vi "Main.vi"(11 "Module Admin":refnum<class "Delacor_lib_QMH_Module Admin.lvclass">) -> ()   [LabVIEW 2024, in "MoneyControl.lvlib"]
doc: "This template is based off of the Queued Message Handler design pattern and the Queued Message Handler project template that ships with LabVIEW.\n\nThe main difference is that the queue is private to this module and communication between modules is performed via Broadcast and Request events.\n\nRequest events are wrapped in public API methods and are handled in the Event Handling Loop (EHL) of this VI. Any module can register for Broadcast events sent by this module. The EHL generates messages based on user interface actions.\n\nThe Message Handling Loop (MHL) processes messages generated by the EHL, or by other messages. The messages are string values, so new messages can be added easily to the Message Cases case structure in the MHL. Each message cluster can also provide an optional value for Message Data, which is a variant that can be converted to whatever message-specific data is required.\n_____\nBased on DQMH Dev Tools: Project Template 7.1.0.1503."
uses:
  MoneyControl.lvlib
  <vilib>/Delacor/Delacor QMH/Libraries/Module Admin_class/Delacor_lib_QMH_Module Admin.lvclass
  Module Data--cluster.ctl
  Incrementa Credito Argument--cluster.ctl
  <vilib>/Delacor/Delacor QMH/Libraries/Message Queue_class/Delacor_lib_QMH_Message Queue.lvclass/Delacor_lib_QMH_Message Queue.ctl
  Stop Argument--cluster.ctl
  <vilib>/Delacor/Delacor QMH/Libraries/Module Admin_class/Delacor_lib_QMH_Module Admin.lvclass/Delacor_lib_QMH_Module Admin.ctl
  Draw FP in Subpanel Argument--cluster.ctl
  Remove From Subpanel Argument--cluster.ctl
  Devuelve dinero Argument--cluster.ctl
  Entrega Cambio Argument--cluster.ctl
  consulta credito Argument--cluster.ctl
  consulta credito (Reply Payload)--cluster.ctl
  <vilib>/Delacor/Delacor QMH/Libraries/Message Queue_class/Delacor_lib_QMH_Enqueue Message (Single).vi
  <vilib>/Delacor/Delacor QMH/Libraries/Module Admin_class/Delacor_lib_QMH_Get External Launch.vi
  <vilib>/Delacor/Delacor QMH/Libraries/Message Queue_class/Delacor_lib_QMH_Message Queue.lvclass
panel:
  in  "1":bool
  out "Status":string
  in  "2":bool
  out "error out":errorcluster
  in  "5":bool
  in  "10":bool
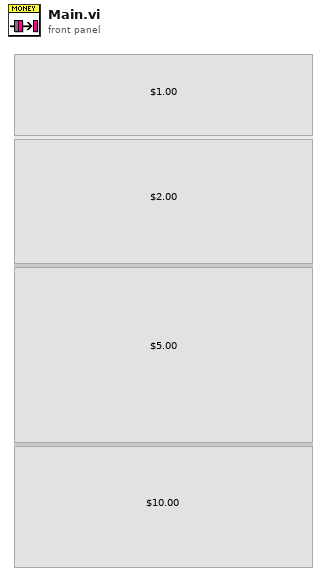
[diagram p1: front panel]
types:
  T1 = typedef "MoneyControl.lvlib/Request Events--cluster.ctl" = cluster{"Stop Module":refnum<user-event>, "Show Panel":refnum<user-event>, "Hide Panel":refnum<user-event>, "Get Module Execution Status":refnum<user-event>, "Show Diagram":refnum<user-event>, "Draw FP in Subpanel":refnum<user-event>, "Remove From Subpanel":refnum<user-event>, "Incrementa Credito":refnum<user-event>, "Devuelve dinero":refnum<user-event>, "Entrega Cambio":refnum<user-event>, "consulta credito":refnum<user-event>}
  T2 = typedef "MoneyControl.lvlib/Module Data--cluster.ctl" = cluster{"Status":string, "Sub Panel":refnum<vi>, "Credito":dbl}
  T3 = typedef "MoneyControl.lvlib/Incrementa Credito Argument--cluster.ctl" = cluster{"Money Value":dbl}
  T4 = enum32{"invalid lock state", "Not Locked", "Locked (No Password)", "Password-protected"}
  T5 = typedef "MoneyControl.lvlib/Stop Argument--cluster.ctl" = cluster{"Origin":string, "Exit via Stop Module Req?":bool, "Wait for Module to stop?":bool}
  T6 = typedef "MoneyControl.lvlib/Draw FP in Subpanel Argument--cluster.ctl" = cluster{"Sub Panel":refnum<vi>}
  T7 = typedef "MoneyControl.lvlib/Remove From Subpanel Argument--cluster.ctl" = cluster{"Boolean":bool}
  T8 = typedef "MoneyControl.lvlib/Devuelve dinero Argument--cluster.ctl" = cluster{"Boolean":bool}
  T9 = typedef "MoneyControl.lvlib/Entrega Cambio Argument--cluster.ctl" = cluster{"Valor Producto":dbl}
  T10 = typedef "MoneyControl.lvlib/consulta credito Argument--cluster.ctl" = cluster{"Wait Notifier":refnum<notifier>, "wait for reply":bool}
  T11 = enum32{"Invalid", "Standard", "Closed", "Hidden", "Minimized", "Maximized"}
  T12 = typedef "MoneyControl.lvlib/consulta credito (Reply Payload)--cluster.ctl" = cluster{"Credito Actual":dbl, "error":errorcluster}
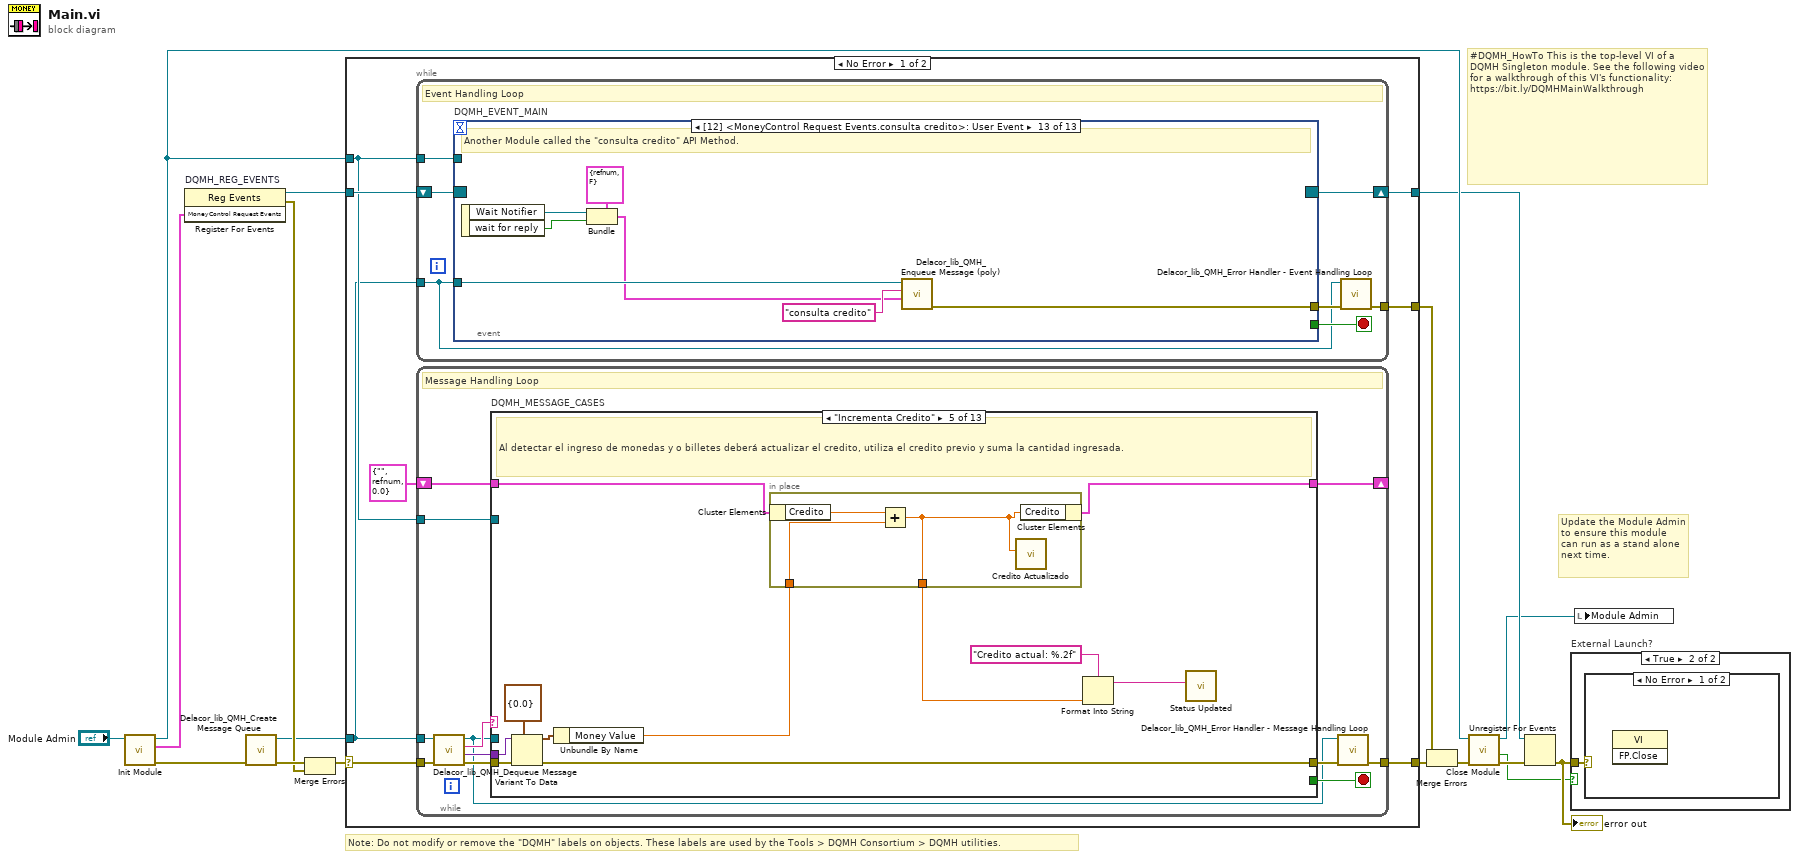
[diagram p0: block diagram]
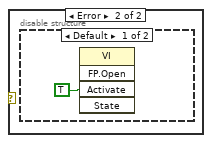
[diagram p3: hidden frame]
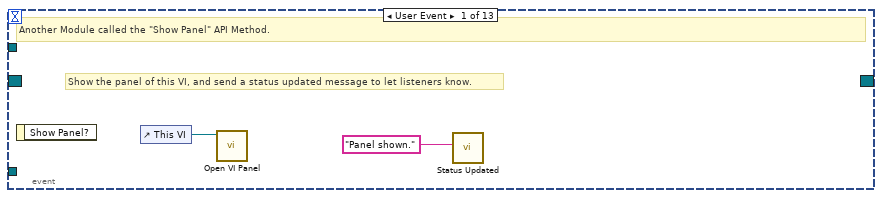
[diagram p5: hidden frame]
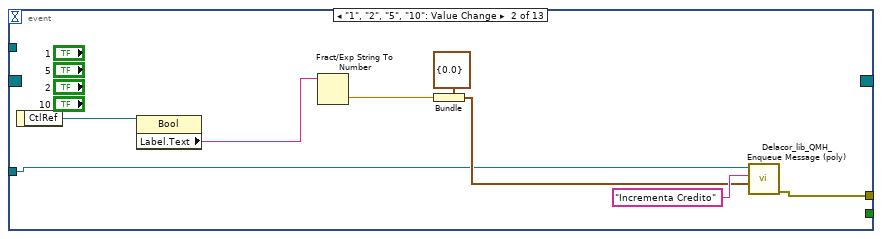
[diagram p6: hidden frame]
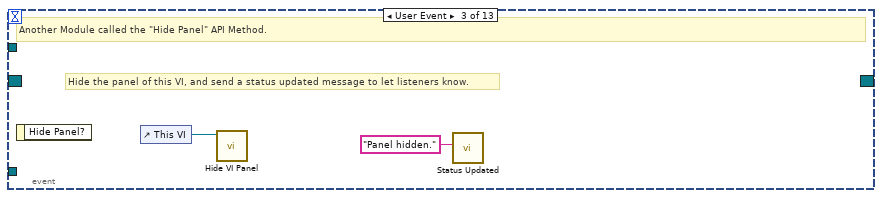
[diagram p7: hidden frame]
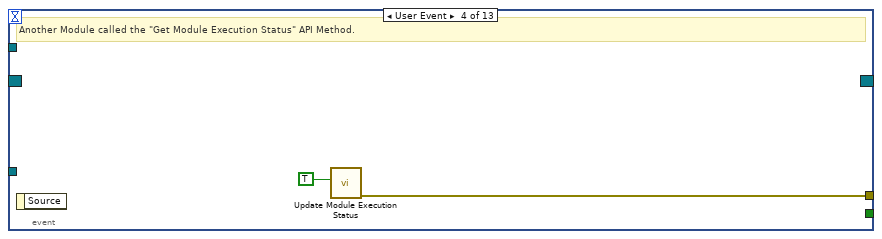
[diagram p8: hidden frame]
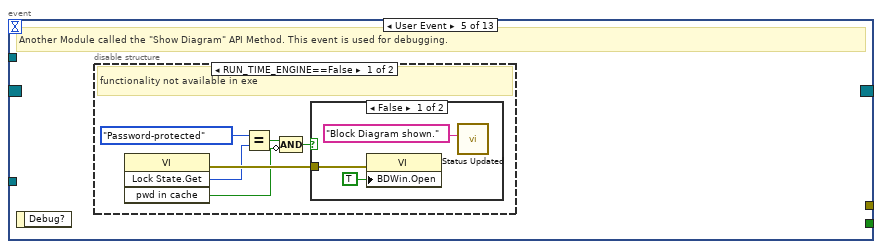
[diagram p9: hidden frame]
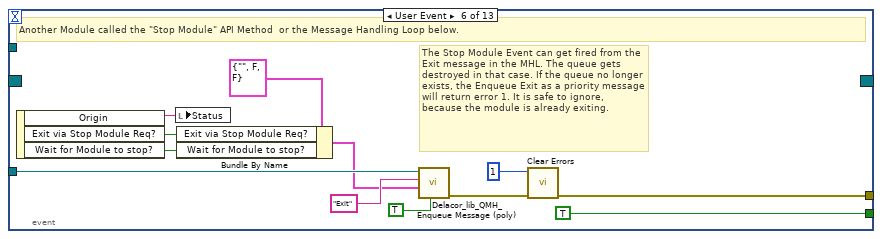
[diagram p12: hidden frame]
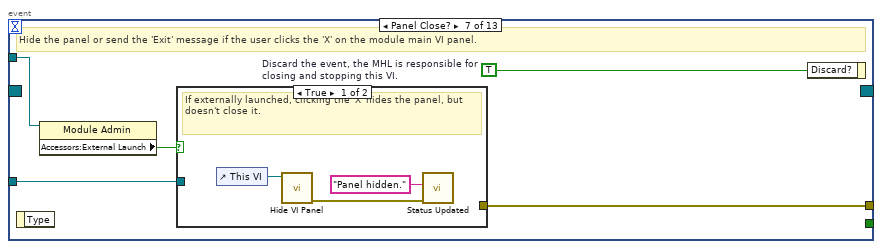
[diagram p13: hidden frame]
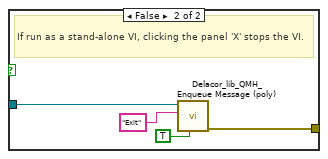
[diagram p14: hidden frame]
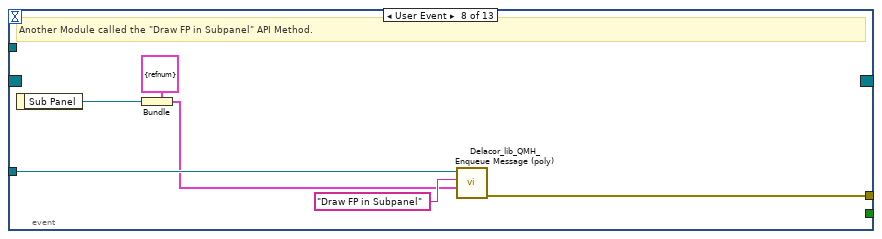
[diagram p15: hidden frame]
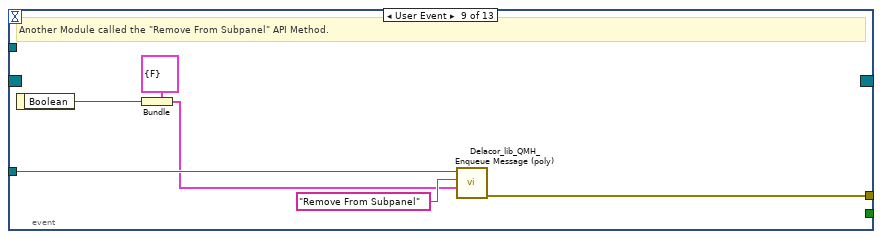
[diagram p16: hidden frame]
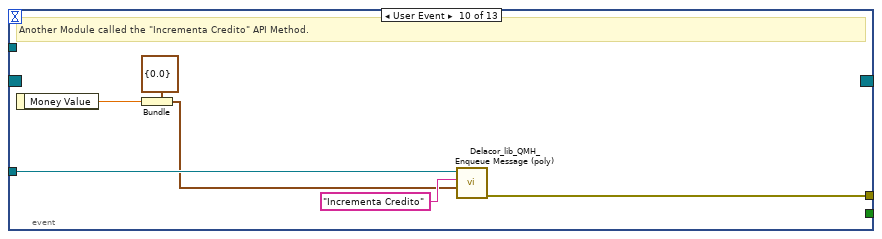
[diagram p17: hidden frame]
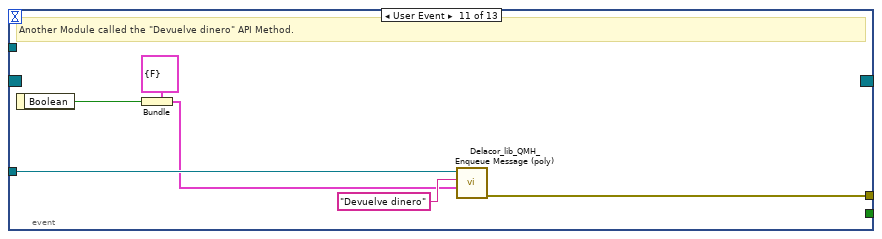
[diagram p18: hidden frame]
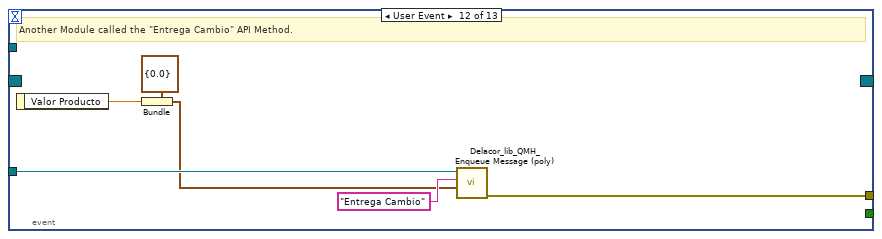
[diagram p19: hidden frame]
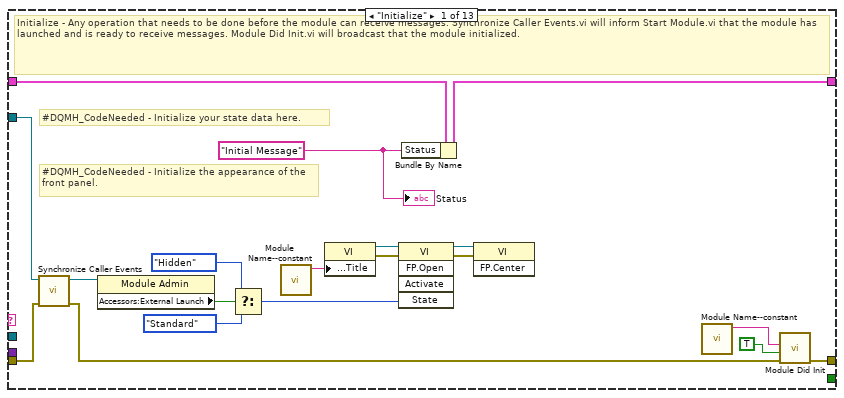
[diagram p20: hidden frame]
diagram:
  # "#DQMH_HowTo This is the top-level VI of a DQMH Singleton module. See the following video for a walkthrough of this VI's functionality: https://bit.ly/DQMHMainWalkthrough"
  # "Note: Do not modify or remove the \"DQMH\" labels on objects. These labels are used by the Tools > DQMH Consortium > DQMH utilities."
  # "Update the Module Admin to ensure this module can run as a stand alone next time."
  n1 = call "Init Module.vi"("Singleton Module Admin in"="Module Admin") -> ("error out"=w16:errorcluster, "MoneyControl Request Events"=w5:T1, "Singleton Module Admin out"=w8:refnum<class "Delacor_lib_QMH_Module Admin.lvclass">)  [unwired: 8 in]
  n2 = register-events "DQMH_REG_EVENTS"(w5) -> (reference out=w6:refnum<event-registration>, error out=w9:errorcluster)  [unwired: 2 in]
  n3 = call <vilib>:"Delacor_lib_QMH_Create Message Queue.vi"("error in"=w16) -> ("error out"=w11:errorcluster, "Message Queue"=w4:refnum<class "Delacor_lib_QMH_Message Queue.lvclass">)  [unwired: 9 in]
  n4 = Merge Errors(w11, w9) -> (w10:errorcluster)
  n5 = case shown="No Error" w10 {
    selector: w10 -> [w23 w296]
    tunnel: [w25 w295] -> w17
    tunnel: [w22 w294] -> w7
    tunnel: w6 -> [w20 w294]
    tunnel: w4 -> [w18 w289]
    tunnel: [w24 _] -> w14
    tunnel: w8 -> [w19 w290]
    frame No Error {
      n6 = while {
        tunnel: w18 -> [w26]
        shift-right: [w29] -> w22
        shift-left: w20 -> [w30]
        tunnel: [w31] -> w24
        tunnel: w19 -> [w27]
        stop <- w28 stop-if-true
        # "Event Handling Loop"
        n7 = event "DQMH_EVENT_MAIN" shown="[12] <MoneyControl Request Events.consulta credito>: User Event" {
          selector: w30 -> [_ _ _ _ _ _ _ _ _ _ _ _ _]
          dyn-events: [_ _ _ _ _ _ _ _ _ _ _ _ _] -> w29
          timeout: _ -> [_ _ _ _ _ _ _ _ _ _ _ _ _]
          tunnel: [_ _ _ _ _ TRUE ("Discard?") _ _ _ _ _ _ _] -> w28
          tunnel: w26 -> [_ w37 _ _ _ w63 w70 w84 w90 w97 w103 w109 w116]
          tunnel: [_ w38 _ w46 _ w66 w72 w85 w91 w92 w98 w104 w110] -> w32
          tunnel: w27 -> [_ _ _ _ _ _ w69 _ _ _ _ _ _]
          event User Event {
            # "Show the panel of this VI, and send a status updated message to let listeners know."
            # "Another Module called the \"Show Panel\" API Method."
            n8 = event-data() -> ()  [unwired: 1 in, 1 out]
            n9 = control-ref of="This VI"() -> (w34:refnum<vi>)
            n10 = call "Open VI Panel.vi"("VI"=w34) -> ()  [unwired: 10 in, 1 out]
            n11 = call "Status Updated.vi"("Status"="Panel shown." ("format string")) -> ()  [unwired: 10 in, 1 out]
          }
          event "1", "2", "5", "10": Value Change {
            n12 = event-data() -> ("CtlRef"=w42:refnum<vi>)  [unwired: 1 in]
            n13 = property class="Bool"(reference=w42) -> ("Label.Text"=w36:string)  [unwired: 1 in, 2 out]
            n14 = Fract/Exp String To Number(string=w36) -> (number=w35:dbl)  [unwired: 3 in, 1 out]
            n15 = Bundle(cluster=T3 {"Money Value"=0.0} ("Incrementa Credito Argument"), "Money Value"=w35) -> (w39:T3)
            n16 = call-poly <vilib>:"Delacor_lib_QMH_Enqueue Message (poly).vi"("Message Data"=w39, "Message"="Incrementa Credito", "Message Queue in"=w37) -> ("error out"=w38:errorcluster)  [unwired: 7 in, 1 out]
          }
          event User Event {
            # "Hide the panel of this VI, and send a status updated message to let listeners know."
            # "Another Module called the \"Hide Panel\" API Method."
            n17 = event-data() -> ()  [unwired: 1 in, 1 out]
            n18 = control-ref of="This VI"() -> (w44:refnum<vi>)
            n19 = call "Hide VI Panel.vi"("VI"=w44) -> ()  [unwired: 10 in, 1 out]
            n20 = call "Status Updated.vi"("Status"="Panel hidden." ("format string")) -> ()  [unwired: 10 in, 1 out]
          }
          event User Event {
            # "Another Module called the \"Get Module Execution Status\" API Method."
            n21 = event-data() -> ()  [unwired: 1 in, 1 out]
            n22 = call "Update Module Execution Status.vi"("Running?"=TRUE) -> ("error out"=w46:errorcluster)  [unwired: 10 in]
          }
          event User Event {
            # "Another Module called the \"Show Diagram\" API Method. This event is used for debugging."
            n23 = event-data() -> ()  [unwired: 1 in, 1 out]
            n24 = disable-structure shown="RUN_TIME_ENGINE==False" {
              frame condition #0 (active) {
                # "functionality not available in exe"
                n25 = invoke on="Invoke Node" class="VI" method="Lock State.Get"() -> (error out=w52:errorcluster, "Get Lock State"=w51:T4, "pwd in cache"=w48:bool)  [unwired: 4 in, 1 out]
                n26 = Equal?(x=T4."Password-protected", y=w51) -> (x = y?=w49:bool)
                n27 = Compound Arithmetic op=AND(w49, invert w48) -> (w47:bool)
                n28 = case shown="False" w47 {
                  tunnel: w52 -> [w55 _]
                  frame False {
                    n29 = property on="Property Node" class="VI"(error in=w55, "BDWin.Open"=TRUE ("Block Diagram Window:Open")) -> ()  [unwired: 1 in, 2 out]
                    n30 = call "Status Updated.vi"("Status"="Block Diagram shown." ("format string")) -> ()  [unwired: 10 in, 1 out]
                  }
                  frame True {
                    # "Password-protected VI, and the password is not in the cache. Do not show the diagram."
                  }
                }
              }
              frame condition #1 {
              }
            }
          }
          event User Event {
            # "The Stop Module Event can get fired from the Exit message in the MHL. The queue gets destroyed in that case. If the queue no longer exists, the Enqueue Exit as a priority message will return error 1. It is safe to ignore, because the module is already exiting."
            # "Another Module called the \"Stop Module\" API Method  or the Message Handling Loop below."
            n31 = event-data() -> ("Origin"=w62:string, "Exit via Stop Module Req?"=w58:bool, "Wait for Module to stop?"=w57:bool)  [unwired: 1 in]
            n32 = local write "Status"(w62) -> ()
            n33 = Bundle By Name(cluster=T5 {"Origin"="", "Exit via Stop Module Req?"=FALSE, "Wait for Module to stop?"=FALSE} ("Stop Argument"), "Exit via Stop Module Req?"=w58, "Wait for Module to stop?"=w57) -> (w56:T5)
            n34 = call-poly <vilib>:"Delacor_lib_QMH_Enqueue Message (poly).vi"("Priority Message? (F)"=TRUE, "Message Data"=w56, "Message"="Exit", "Message Queue in"=w63) -> ("error out"=w67:errorcluster)  [unwired: 6 in, 1 out]
            n35 = call <vilib>:"Clear Errors.vi"("error in (no error)"=w67, "specific error code to clear (0: all)"=1) -> ("error out"=w66:errorcluster)  [unwired: 4 in, 1 out]
          }
          event Panel Close? {
            w71 = TRUE  # Discard the event, the MHL is responsible for closing and stopping this VI.
            # "Hide the panel or send the 'Exit' message if the user clicks the 'X' on the module main VI panel."
            n36 = event-data() -> ()  [unwired: 1 in, 1 out]
            n37 = property on="Property Node" class="Module Admin"(reference=w69) -> ("Accessors:External Launch"=w68:bool)  [unwired: 1 in, 2 out]
            n38 = case shown="True" w68 {
              tunnel: w70 -> [_ w78]
              tunnel: [_ w79] -> w72
              frame True {
                # "If externally launched, clicking the 'X' hides the panel, but doesn't close it."
                n39 = control-ref of="This VI"() -> (w74:refnum<vi>)
                n40 = call "Hide VI Panel.vi"("VI"=w74) -> ("error out"=w75:errorcluster)  [unwired: 10 in]
                n41 = call "Status Updated.vi"("error in"=w75, "Status"="Panel hidden." ("format string")) -> ()  [unwired: 9 in, 1 out]
              }
              frame False {
                # "If run as a stand-alone VI, clicking the panel 'X' stops the VI."
                n42 = call-poly <vilib>:"Delacor_lib_QMH_Enqueue Message (poly).vi"("Priority Message? (F)"=TRUE, "Message"="Exit", "Message Queue in"=w78) -> ("error out"=w79:errorcluster)  [unwired: 7 in, 1 out]
              }
            }
            n43 = event-data ("Event Filter Node")("Discard?"=w71) -> ()  [unwired: 1 in, 1 out]
          }
          event User Event {
            # "Another Module called the \"Draw FP in Subpanel\" API Method."
            n44 = event-data() -> ("Sub Panel"=w80:refnum<vi>)  [unwired: 1 in]
            n45 = Bundle(cluster=T6 {"Sub Panel"=refnum} ("Draw FP in Subpanel Argument"), "Sub Panel"=w80) -> (w81:T6)
            n46 = call-poly <vilib>:"Delacor_lib_QMH_Enqueue Message (poly).vi"("Message Data"=w81, "Message"="Draw FP in Subpanel", "Message Queue in"=w84) -> ("error out"=w85:errorcluster)  [unwired: 7 in, 1 out]
          }
          event User Event {
            # "Another Module called the \"Remove From Subpanel\" API Method."
            n47 = event-data() -> ("Boolean"=w86:bool)  [unwired: 1 in]
            n48 = Bundle(cluster=T7 {"Boolean"=FALSE} ("Remove From Subpanel Argument"), "Boolean"=w86) -> (w87:T7)
            n49 = call-poly <vilib>:"Delacor_lib_QMH_Enqueue Message (poly).vi"("Message Data"=w87, "Message"="Remove From Subpanel", "Message Queue in"=w90) -> ("error out"=w91:errorcluster)  [unwired: 7 in, 1 out]
          }
          event User Event {
            # "Another Module called the \"Incrementa Credito\" API Method."
            n50 = event-data() -> ("Money Value"=w93:dbl)  [unwired: 1 in]
            n51 = Bundle(cluster=T3 {"Money Value"=0.0} ("Incrementa Credito Argument"), "Money Value"=w93) -> (w94:T3)
            n52 = call-poly <vilib>:"Delacor_lib_QMH_Enqueue Message (poly).vi"("Message Data"=w94, "Message"="Incrementa Credito", "Message Queue in"=w97) -> ("error out"=w92:errorcluster)  [unwired: 7 in, 1 out]
          }
          event User Event {
            # "Another Module called the \"Devuelve dinero\" API Method."
            n53 = event-data() -> ("Boolean"=w99:bool)  [unwired: 1 in]
            n54 = Bundle(cluster=T8 {"Boolean"=FALSE} ("Devuelve dinero Argument"), "Boolean"=w99) -> (w100:T8)
            n55 = call-poly <vilib>:"Delacor_lib_QMH_Enqueue Message (poly).vi"("Message Data"=w100, "Message"="Devuelve dinero", "Message Queue in"=w103) -> ("error out"=w98:errorcluster)  [unwired: 7 in, 1 out]
          }
          event User Event {
            # "Another Module called the \"Entrega Cambio\" API Method."
            n56 = event-data() -> ("Valor Producto"=w105:dbl)  [unwired: 1 in]
            n57 = Bundle(cluster=T9 {"Valor Producto"=0.0} ("Entrega Cambio Argument"), "Valor Producto"=w105) -> (w106:T9)
            n58 = call-poly <vilib>:"Delacor_lib_QMH_Enqueue Message (poly).vi"("Message Data"=w106, "Message"="Entrega Cambio", "Message Queue in"=w109) -> ("error out"=w104:errorcluster)  [unwired: 7 in, 1 out]
          }
          event User Event {
            # "Another Module called the \"consulta credito\" API Method."
            n59 = event-data() -> ("Wait Notifier"=w112:refnum<notifier>, "wait for reply"=w111:bool)  [unwired: 1 in]
            n60 = Bundle(cluster=T10 {"Wait Notifier"=refnum, "wait for reply"=FALSE} ("consulta credito Argument"), "Wait Notifier"=w112, "wait for reply"=w111) -> (w113:T10)
            n61 = call-poly <vilib>:"Delacor_lib_QMH_Enqueue Message (poly).vi"("Message Data"=w113, "Message"="consulta credito", "Message Queue in"=w116) -> ("error out"=w110:errorcluster)  [unwired: 7 in, 1 out]
          }
        }
        n62 = call-dynamic "Delacor_lib_QMH_Error Handler - Event Handling Loop.vi"("error in"=w32, "Message Queue in"=w26) -> ("dup error in"=w31:errorcluster)  [unwired: 8 in, 1 out]
      }
      n63 = while {
        tunnel: w18 -> [w117]
        shift-right: [w123] -> _
        shift-left: T2 {"Status"="", "Sub Panel"=refnum, "Credito"=0.0} ("Data Cluster") -> [w124]
        tunnel: w23 -> [w128]
        tunnel: [w126] -> w25
        tunnel: w19 -> [w119]
        stop <- w122 stop-if-true
        # "Message Handling Loop"
        n64 = call-dynamic "Delacor_lib_QMH_Dequeue Message.vi"("error in"=w128, "Message Queue in"=w117) -> ("error out"=w127:errorcluster, "Message Data"=w120:variant, "Message"=w121:string, "Message Queue out"=w118:refnum<class "Delacor_lib_QMH_Message Queue.lvclass">)  [unwired: 6 in]
        n65 = case "DQMH_MESSAGE_CASES" shown="\"Incrementa Credito\"" w121 {
          selector: w121 -> [_ _ _ _ _ _ _ _ _ _ _ _ w284]
          tunnel: w118 -> [_ _ _ _ _ _ _ _ _ _ w248 w272 _]
          tunnel: w127 -> [w145 w149 w165 w183 w200 w214 w222 w238 w243 w245 w256 w278 w287]
          tunnel: [w143 w149 w164 w181 w199 w213 w221 w229 w242 w245 w252 w273 w288] -> w125
          tunnel: w124 -> [w134 w148 w160 w177 w195 w208 w217 w228 w241 w244 w250 w264 w285]
          tunnel: [w133 w148 w156 w174 w194 w209 w216 w228 w241 w244 w250 w264 w285] -> w123
          tunnel: [_ _ _ _ _ _ _ _ _ _ _ w271 _] -> w122
          tunnel: w120 -> [_ _ w159 w180 w198 w212 w220 w236 _ _ w249 w270 _]
          tunnel: w119 -> [w135 _ _ _ _ _ _ _ _ _ w247 w265 _]
          frame "Initialize" {
            w129 = "Initial Message" ("Initial Message")
            # "#DQMH_CodeNeeded - Initialize the appearance of the front panel."
            # "#DQMH_CodeNeeded - Initialize your state data here."
            # "Initialize - Any operation that needs to be done before the module can receive messages. Synchronize Caller Events.vi will inform Start Module.vi that the module has launched and is ready to receive messages. Module Did Init.vi will broadcast that the module initialized."
            n66 = call "Synchronize Caller Events.vi"("error in"=w145, "Singleton Module Admin in"=w135) -> ("error out"=w144:errorcluster, "Singleton Module Admin out"=w130:refnum<class "Delacor_lib_QMH_Module Admin.lvclass">)  [unwired: 8 in]
            n67 = property on="Property Node" class="Module Admin"(reference=w130) -> ("Accessors:External Launch"=w139:bool)  [unwired: 1 in, 2 out]
            n68 = Select(t=T11."Hidden" ("State"), s=w139, f=T11."Standard" ("State")) -> (s? t:f=w136:T11)
            n69 = call "Module Name--constant.vi"() -> ("Module Name"=w142:string)  [unwired: 11 in]
            n70 = property on="Property Node" class="VI"("Front Panel.Title"=w142) -> (reference out=w141:refnum<vi>, error out=w147:errorcluster)  [unwired: 2 in]
            n71 = invoke on="Invoke Node" class="VI" method="FP.Open"(reference=w141, error in=w147, "State"=w136) -> (reference out=w140:refnum<vi>, error out=w146:errorcluster)  [unwired: 2 in, 3 out]
            n72 = Bundle By Name(cluster=w134, "Status"=w129) -> (w133:T2)
            n73 = invoke on="Invoke Node" class="VI" method="FP.Center"(reference=w140, error in=w146) -> ()  [unwired: 1 in, 3 out]
            n74 = call "Module Name--constant.vi"() -> ("Module Name"=w131:string)  [unwired: 11 in]
            n75 = call "Module Did Init.vi"("error in"=w144, "Initialized?"=TRUE, "Origin"=w131) -> ("error out"=w143:errorcluster)  [unwired: 8 in]
            "Status" <- w129
          }
          frame "---Module Specific---" {
            # "Separator -- The following cases handle messages specific to this Module."
          }
          frame "Draw FP in Subpanel" {
            # "Draw FP in Subpanel"
            n76 = Variant To Data(error in=w165, type=T6 {"Sub Panel"=refnum} ("Draw FP in Subpanel Argument"), Variant=w159) -> (data=w157:T6, error out=w163:errorcluster)
            n77 = Unbundle By Name(w157) -> ("Sub Panel"=w155:refnum<vi>)
            n78 = control-ref of="This VI"() -> (w152:refnum<vi>)
            n79 = property class="VI"(reference=w152, error in=w163) -> (reference out=w151:refnum<vi>, error out=w161:errorcluster, "FP.State"=w150:T11)
            n80 = case shown="\"Closed\"" w150 {
              tunnel: [w166 w169] -> w153
              tunnel: [w167 w171] -> w162
              tunnel: w161 -> [w167 w170]
              tunnel: w151 -> [w166 w168]
              frame "Closed" {
              }
              frame "Standard", Default {
                n81 = invoke class="VI" method="FP.Close"(reference=w168, error in=w170) -> (reference out=w169:refnum<vi>, error out=w171:errorcluster)  [unwired: 1 in, 1 out]
              }
            }
            n82 = invoke class="SubPnl" method="Insert VI"(reference=w155, error in=w162, "VI Ref"=w153) -> (reference out=w154:refnum<vi>, error out=w164:errorcluster)  [unwired: 1 in, 2 out]
            n83 = Bundle By Name(cluster=w160, "Sub Panel"=w154) -> (w156:T2)
          }
          frame "Remove From Subpanel" {
            # "Remove From Subpanel"
            n84 = Variant To Data(error in=w183, type=T7 {"Boolean"=FALSE} ("Remove From Subpanel Argument"), Variant=w180) -> (data=w178:T7, error out=w182:errorcluster)
            n85 = Unbundle By Name(w178) -> ()  [unwired: 1 out]
            n86 = Unbundle By Name(w177) -> ("Sub Panel"=w176:refnum<vi>)
            n87 = Not A Number/Path/Refnum?(number/path/refnum=w176) -> (NaN/Path/Refnum?=w175:bool)
            n88 = case shown="True" w175 {
              tunnel: w182 -> [w187 w189]
              tunnel: [w186 w189] -> w181
              tunnel: w176 -> [w185 _]
              tunnel: ["Module Removed from Subpanel" "This module has not been inserted into the subpanel"] -> w172
              frame False {
                n89 = invoke class="SubPnl" method="Remove VI"(reference=w185, error in=w187) -> (error out=w186:errorcluster)  [unwired: 1 in, 2 out]
              }
              frame True {
              }
            }
            n90 = Bundle By Name(cluster=w177, "Sub Panel"=refnum<vi> refnum) -> (w174:T2)
            n91 = call "Status Updated.vi"("Status"=w172) -> ()  [unwired: 10 in, 1 out]
          }
          frame "Incrementa Credito" {
            # "Al detectar el ingreso de monedas y o billetes deberá actualizar el credito, utiliza el credito previo y suma la cantidad ingresada."
            n92 = Variant To Data(error in=w200, type=T3 {"Money Value"=0.0} ("Incrementa Credito Argument"), Variant=w198) -> (data=w196:T3, error out=w199:errorcluster)
            n93 = Unbundle By Name(w196) -> ("Money Value"=w193:dbl)
            n94 = in-place {
              in-place-border: w193 -> [w202]
              in-place-border: [w201] -> w191
              n95 = in-place-cluster #1(w195) -> ("Credito"=w203:dbl)
              n96 = Add(x=w203, y=w202) -> (x+y=w201:dbl)
              n97 = call "Credito Actualizado.vi"("Credito"=w201) -> ()  [unwired: 10 in, 1 out]
              n98 = in-place-cluster #1("Credito"=w201) -> (w194:T2)
            }
            n99 = Format Into String(format string="Credito actual: %.2f", w191) -> (resulting string=w192:string)  [unwired: 2 in, 1 out]
            n100 = call "Status Updated.vi"("Status"=w192) -> ()  [unwired: 10 in, 1 out]
          }
          frame "Devuelve dinero" {
            w206 = 0.0 ("Credito")
            # "Esta accion es la de cancelar la compra"
            n101 = Variant To Data(error in=w214, type=T8 {"Boolean"=FALSE} ("Devuelve dinero Argument"), Variant=w212) -> (data=w210:T8, error out=w213:errorcluster)
            n102 = Unbundle By Name(w210) -> ()  [unwired: 1 out]
            n103 = Unbundle By Name(w208) -> ("Credito"=w205:dbl)
            n104 = call "Cambio Actualizado.vi"("Cambio"=w205) -> ()  [unwired: 10 in, 1 out]
            n105 = call "Credito Actualizado.vi"("Credito"=w206) -> ()  [unwired: 10 in, 1 out]
            n106 = Bundle By Name(cluster=w208, "Credito"=w206) -> (w209:T2)
            n107 = Format Into String(format string="Devolviendo dinero: Credito Actual%.2f, Cambio: %.2f", w206, w205) -> (resulting string=w207:string)  [unwired: 2 in, 1 out]
            n108 = call "Status Updated.vi"("Status"=w207) -> ()  [unwired: 10 in, 1 out]
          }
          frame "Entrega Cambio" {
            # "Request para entregar cambio despues de hacer venta"
            n109 = Variant To Data(error in=w222, type=T9 {"Valor Producto"=0.0} ("Entrega Cambio Argument"), Variant=w220) -> (data=w218:T9, error out=w221:errorcluster)
            n110 = Unbundle By Name(w218) -> ("Valor Producto"=w215:dbl)
            n111 = in-place {
              in-place-border: w215 -> [w225]
              w224 = 0.0 ("Credito")
              n112 = in-place-cluster #2(w217) -> ("Credito"=w226:dbl)
              n113 = Subtract(x=w226, y=w225) -> (x-y=w223:dbl)
              n114 = call "Cambio Actualizado.vi"("Cambio"=w223) -> ()  [unwired: 10 in, 1 out]
              n115 = call "Credito Actualizado.vi"("Credito"=w224) -> ()  [unwired: 10 in, 1 out]
              n116 = in-place-cluster #2("Credito"=w224) -> (w216:T2)
            }
          }
          frame "consulta credito" {
            n117 = Variant To Data(error in=w238, type=T10 {"Wait Notifier"=refnum, "wait for reply"=FALSE} ("consulta credito Argument"), Variant=w236) -> (data=w234:T10, error out=w237:errorcluster)
            n118 = Unbundle By Name(w234) -> ("Wait Notifier"=w233:refnum<notifier>, "wait for reply"=w232:bool)
            n119 = Unbundle By Name(w228) -> ("Credito"=w227:dbl)
            n120 = Bundle By Name(cluster=T12 {"Credito Actual"=0.0, "error"={"status"=FALSE, "code"=0, "source"=""}} ("consulta credito (Reply Payload)"), "Credito Actual"=w227) -> (w231:T12)
            n121 = Merge Errors(w237) -> (w229:errorcluster)
            n122 = case "DQMH_FIRE_NOTIFIER" shown="True" w232 {
              tunnel: w233 -> [_ w240]
              tunnel: w231 -> [_ w239]
              frame False {
              }
              frame True {
                n123 = Send Notification(notification=w239, notifier=w240) -> ()  [unwired: 1 in, 2 out]
              }
            }
          }
          frame "---Copy This Frame---" {
            # "Duplicate this frame when creating new messages.  Change this comment in the duplicated frame to describe this message."
            n124 = Merge Errors(w243) -> (w242:errorcluster)
          }
          frame "---Exit and Error Handling---" {
            # "Separator - The following cases handle errors and exit messages."
          }
          frame "Error" {
            # "#DQMH_CodeRecommended - If the module is running in standalone mode (External Launch = FALSE), this code will pop up an error dialog and call the 'Exit' message if an error occurs. Add more fine-grained error management here."
            # "Error - Check the error message data and respond accordingly. This message is sent by the \"Error Handler\" VIs at the end of each loop in this application."
            n125 = property on="Property Node" class="Module Admin"(reference=w247) -> ("Accessors:External Launch"=w246:bool)  [unwired: 1 in, 2 out]
            n126 = Variant To Data(error in=w256, type=errorcluster {"status"=FALSE, "code"=0, "source"=""} ("error constant"), Variant=w249) -> (data=w251:errorcluster, error out=w254:errorcluster)
            n127 = local write "error out"(w251) -> ()
            n128 = call "Error Reported.vi"("Error"=w251) -> ()  [unwired: 10 in, 1 out]
            n129 = case shown="False" w246 {
              tunnel: [w261 _] -> w253
              tunnel: w248 -> [w259 _]
              tunnel: w251 -> [w260 _]
              frame False {
                n130 = disable-structure shown="Default" {
                  disable-tunnel: w260 -> [w262 _]
                  frame condition #0 (active) {
                    # "If the module is running standalone, then pop up an error dialog and call the \"Exit\" message."
                    n131 = call <vilib>:"Simple Error Handler.vi"("error in (no error)"=w262) -> ()  [unwired: 4 in, 5 out]
                  }
                  frame condition #1 {
                    # "To prevent the Simple Error Handler VI from being loaded (e.g. when deploying to a Real-Time target), add the Conditional Disable Symbol \"DQMH_Disable_SEH\" to your project and set it to TRUE."
                  }
                }
                n132 = call-poly <vilib>:"Delacor_lib_QMH_Enqueue Message (poly).vi"("Priority Message? (F)"=TRUE, "Message"="Exit", "Message Queue in"=w259) -> ("error out"=w261:errorcluster)  [unwired: 7 in, 1 out]
              }
              frame True {
                # "If the module was launched externally, calling the Error Reported broadcast VI is the only action performed by the \"Error\" message. The module's caller can then process the error appropriately."
              }
            }
            n133 = Merge Errors(w254, w253) -> (w252:errorcluster)
          }
          frame "Exit" {
            w269 = 91  # 91: not all Exit messages will have an argument
            w271 = TRUE  # Stop the VI
            # "Release the message queue reference"
            # "#DQMH_CodeNeeded - Add any required cleanup code here."
            # "Exit - Exit the application."
            n134 = Variant To Data(error in=w278, type=T5 {"Origin"="", "Exit via Stop Module Req?"=FALSE, "Wait for Module to stop?"=FALSE} ("Stop Argument"), Variant=w270) -> (data=w267:T5, error out=w275:errorcluster)
            n135 = call <vilib>:"Clear Errors.vi"("error in (no error)"=w275, "specific error code to clear (0: all)"=w269) -> ("error out"=w277:errorcluster)  [unwired: 4 in, 1 out]
            n136 = control-ref of="This VI"() -> (w266:refnum<vi>)
            n137 = call-dynamic "Delacor_lib_QMH_Release Message Queue.vi"("error in"=w277, "Message Queue"=w272) -> ("error out"=w276:errorcluster)  [unwired: 9 in]
            n138 = call "Handle Exit.vi"("Stop Argument"=w267, "Admin in"=w265, "VI reference"=w266) -> ("error out"=w274:errorcluster)  [unwired: 7 in, 1 out]
            n139 = Merge Errors(w276, w274) -> (w273:errorcluster)
            n140 = Unbundle By Name(w264) -> ("Sub Panel"=w263:refnum<vi>)
            n141 = call "Error Reported.vi"("Error"=w273) -> ()  [unwired: 10 in, 1 out]
            n142 = invoke class="SubPnl" method="Remove VI"(reference=w263) -> ()  [unwired: 2 in, 3 out]
          }
          frame Default {
            # "'Default' case only runs if there is a message that isn't defined in any of the other cases.  Output a programming error."
            n143 = call "Module Name--constant.vi"() -> ("Module Name"=w283:string)  [unwired: 11 in]
            n144 = Format Into String(format string="The invalid message string \"%s\" was received in the Message Handling Loop for module \"%s\".", w284, w283) -> (resulting string=w279:string)  [unwired: 2 in, 1 out]
            n145 = call <vilib>:"Error Cluster From Error Code.vi"("show call chain? (False)"=TRUE, "error message (\"\")"=w279, "error code (0)"=1) -> ("error out"=w286:errorcluster)  [unwired: 6 in]
            n146 = Merge Errors(w287, w286) -> (w288:errorcluster)
          }
        }
        n147 = call-dynamic "Delacor_lib_QMH_Error Handler - Message Handling Loop.vi"("error in"=w125, "Message Queue in"=w118) -> ("dup error in"=w126:errorcluster)  [unwired: 8 in, 1 out]
      }
    }
    frame Error {
      # "Synchronize Caller Events.vi will inform Start Module.vi that the module has launched and will let the code calling Start Module.vi register for broadcasts and would permit the caller receive the broadcast that an error occurred at launch time."
      n148 = call-dynamic "Delacor_lib_QMH_Release Message Queue.vi"("error in"=w296, "Message Queue"=w289) -> ("error out"=w295:errorcluster)  [unwired: 9 in]
      n149 = call "Synchronize Caller Events.vi"("Singleton Module Admin in"=w290) -> ("error out"=w297:errorcluster)  [unwired: 9 in, 1 out]
      n150 = call "Module Name--constant.vi"() -> ("Module Name"=w293:string)  [unwired: 11 in]
      n151 = Format Into String(format string="An error occurred during initialization. %s is no longer running.", w293) -> (resulting string=w291:string)  [unwired: 2 in, 1 out]
      n152 = Merge Errors(w295, w297) -> (w298:errorcluster)
      n153 = call "Error Reported.vi"("Additional Information"=w291, "Error"=w298) -> ()  [unwired: 9 in, 1 out]
    }
  }
  n154 = Merge Errors(w14, w17) -> (w13:errorcluster)
  n155 = call "Close Module.vi"("error in"=w13, "Module Admin in"=w8) -> ("error out"=w15:errorcluster, "External Launch"=w1:bool, "Module Admin out"=w2:refnum<class "Delacor_lib_QMH_Module Admin.lvclass">)  [unwired: 7 in]
  n156 = Unregister For Events(event registration refnum=w7, error in=w15) -> (error out=w12:errorcluster)
  "error out" <- w12
  n157 = case "External Launch?" shown="True" w1 {
    tunnel: w12 -> [_ w299]
    frame False {
    }
    frame True {
      n158 = case shown="No Error" w299 {
        frame No Error {
          n159 = invoke on="Invoke Node" class="VI" method="FP.Close"() -> ()  [unwired: 3 in, 3 out]
        }
        frame Error {
          n160 = disable-structure shown="Default" {
            frame condition #0 (active) {
              n161 = invoke class="VI" method="FP.Open"("Activate"=TRUE ("Activate?")) -> ()  [unwired: 4 in, 5 out]
            }
            frame condition #1 {
              # "Don't show panel on error if running inside a built EXE."
            }
          }
        }
      }
    }
  }
  n162 = local write "Module Admin"(w2) -> ()
